vi "LV_client.vi"() -> ()   [LabVIEW 2020]
panel:
  out "Path to server Python script":path
  out "error out":errorcluster
  in  "Stop":bool
  out "Answer":string
  in  "Ping":bool
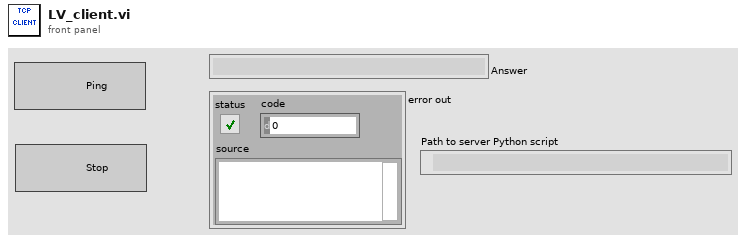
[diagram p1: front panel]
types:
  T1 = enum8{"Enabled", "Disabled", "Disabled and Grayed Out"}
  T2 = enum16{"Standard", "Buffered", "CRLF", "Immediate"}
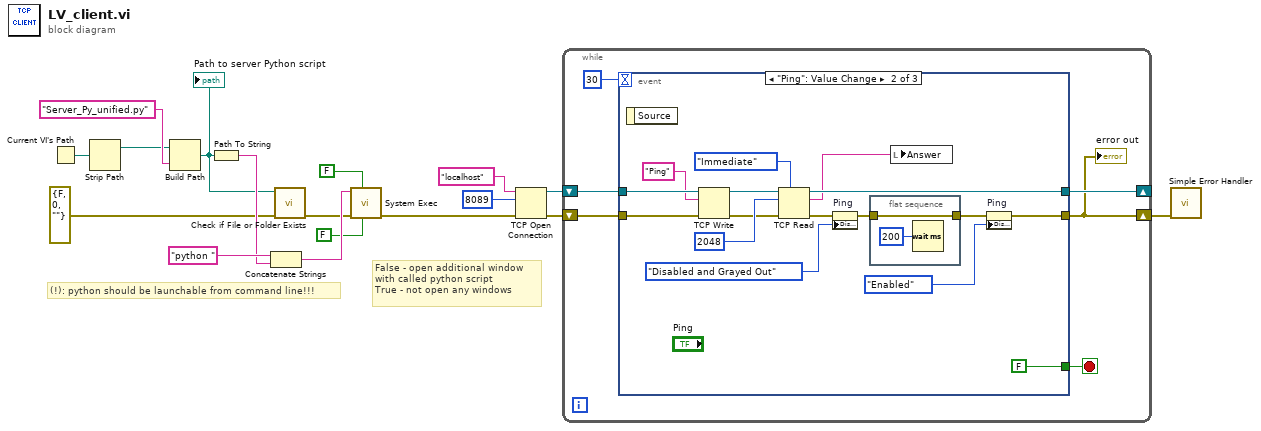
[diagram p0: block diagram]
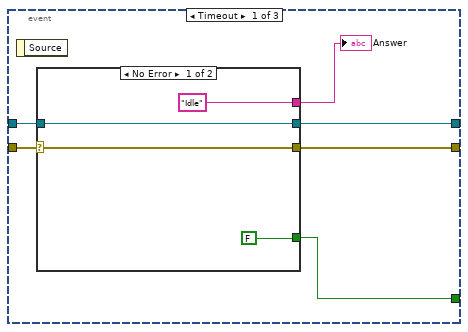
[diagram p2: hidden frame]
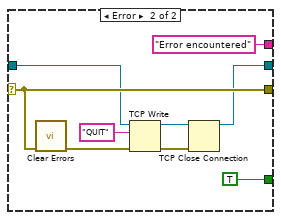
[diagram p3: hidden frame]
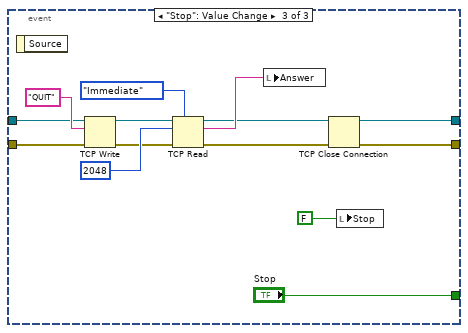
[diagram p4: hidden frame]
diagram:
  # "False - open additional window\nwith called python script\nTrue - not open any windows"
  # "(!): python should be launchable from command line!!!"
  n1 = Current VI's Path() -> (path=w12:path)
  n2 = Strip Path(path=w12) -> (stripped path=w5:path)  [unwired: 1 out]
  n3 = Build Path(base path=w5, name or relative path="Server_Py_unified.py" ("string")) -> (appended path=w3:path)
  "Path to server Python script" <- w3
  n4 = Path To String(path=w3) -> (string=w6:string)
  n5 = Concatenate Strings("python " ("command line"), w6) -> (w10:string)
  n6 = call <vilib>:"Check if File or Folder Exists.vi"("error in (no error)"=errorcluster {"status"=FALSE, "code"=0, "source"=""}, "path"=w3) -> ("error out"=w2:errorcluster)  [unwired: 7 in, 2 out]
  n7 = call <vilib>:"System Exec.vi"("run minimized? (F)"=FALSE, "wait until completion? (T)"=FALSE, "error in (no error)"=w2, "command line"=w10) -> ("error out"=w9:errorcluster)  [unwired: 4 in, 3 out]
  n8 = TCP Open Connection(address="localhost", remote port or service name=u16 8089, error in (no error)=w9) -> (connection ID=w16:refnum<k5>, error out=w15:errorcluster)  [unwired: 2 in]
  n9 = while {
    shift-right: [w20] -> _
    shift-left: w16 -> [w21]
    shift-right: [w18] -> w13
    shift-left: w15 -> [w22]
    stop <- w19 stop-if-true
    n10 = event shown="[1] \"Ping\": Value Change" {
      selector: _ -> [_ _ _]
      dyn-events: _ -> [_ _ _]
      timeout: 30 -> [_ _ _]
      tunnel: [w25 FALSE ("Stop") "Stop"] -> w19
      tunnel: w22 -> [w29 w57 w68]
      tunnel: w21 -> [w28 w58 w67]
      tunnel: [w27 w51 w62] -> w20
      tunnel: [w26 w44 w61] -> w18
      event Timeout {
        n11 = event-data() -> ()  [unwired: 1 in, 1 out]
        n12 = case shown="No Error" w29 {
          selector: w29 -> [w32 w39]
          tunnel: [w33 w35] -> w27
          tunnel: w28 -> [w33 w38]
          tunnel: [w32 w39] -> w26
          tunnel: [FALSE ("Stop") TRUE ("Stop")] -> w25
          tunnel: ["Idle" ("Answer") "Error encountered" ("Answer")] -> w24
          frame No Error {
          }
          frame Error {
            n13 = call <vilib>:"Clear Errors.vi"("error in (no error)"=w39) -> ("error out"=w42:errorcluster)  [unwired: 5 in, 1 out]
            n14 = TCP Write(connection ID=w38, data in="QUIT", error in (no error)=w42) -> (connection ID out=w36:refnum<k5>, error out=w37:errorcluster)  [unwired: 1 in, 1 out]
            n15 = TCP Close Connection(connection ID=w36, error in (no error)=w37) -> (connection ID out=w35:refnum<k5>)  [unwired: 1 in, 1 out]
          }
        }
        "Answer" <- w24
      }
      event "Ping": Value Change {
        n16 = event-data() -> ()  [unwired: 1 in, 1 out]
        n17 = TCP Write(connection ID=w58, data in="Ping", error in (no error)=w57) -> (connection ID out=w55:refnum<k5>, error out=w52:errorcluster)  [unwired: 1 in, 1 out]
        n18 = TCP Read(connection ID=w55, bytes to read=2048, error in (no error)=w52, 7:T2."Immediate" ("mode (standard)")) -> (connection ID out=w51:refnum<k5>, data out=w49:string, error out=w48:errorcluster)  [unwired: 1 in]
        n19 = property on="Ping" class="Bool"(error in=w48, "DisabledEnum"=T1."Disabled and Grayed Out" ("Disabled")) -> (error out=w47:errorcluster)  [unwired: 1 in, 1 out]
        n20 = flat-sequence {
          tunnel: w47 -> [w59]
          tunnel: [w59] -> w45
          frame #0 {
            n21 = Wait (ms)(milliseconds to wait=u32 200) -> ()  [unwired: 1 out]
          }
        }
        n22 = local write "Answer"(w49) -> ()
        n23 = property on="Ping" class="Bool"(error in=w45, "DisabledEnum"=T1."Enabled" ("Disabled")) -> (error out=w44:errorcluster)  [unwired: 1 in, 1 out]
      }
      event "Stop": Value Change {
        n24 = event-data() -> ()  [unwired: 1 in, 1 out]
        n25 = TCP Write(connection ID=w67, data in="QUIT", error in (no error)=w68) -> (connection ID out=w72:refnum<k5>, error out=w69:errorcluster)  [unwired: 1 in, 1 out]
        n26 = TCP Read(connection ID=w72, bytes to read=2048, error in (no error)=w69, 7:T2."Immediate" ("mode (standard)")) -> (connection ID out=w63:refnum<k5>, data out=w66:string, error out=w64:errorcluster)  [unwired: 1 in]
        n27 = local write "Answer"(w66) -> ()
        n28 = TCP Close Connection(connection ID=w63, error in (no error)=w64) -> (connection ID out=w62:refnum<k5>, error out=w61:errorcluster)  [unwired: 1 in]
        n29 = local write "Stop"(FALSE ("Stop")) -> ()
      }
    }
    "error out" <- w18
  }
  n30 = call <vilib>:"Simple Error Handler.vi"("error in (no error)"=w13) -> ()  [unwired: 4 in, 5 out]
